vi "FRC-TrajLib-geometry-sample.vi"() -> ()   [LabVIEW 2019]
uses:
  _misc/ROBOT_PICTURE.ctl
  <vilib>/Rock Robotics/WPI/ThirdParty/JAS_Junk/TrajLib/POSE2D.ctl
  <vilib>/Rock Robotics/WPI/ThirdParty/JAS_Junk/TrajLib/TRANSLATION2D.ctl
  <vilib>/Rock Robotics/WPI/ThirdParty/JAS_Junk/TrajLib/ROTATION2D.ctl
  <vilib>/Rock Robotics/WPI/ThirdParty/JAS_Junk/TrajLib/Rotation2d_CreateAngle.vi
  <vilib>/Rock Robotics/WPI/ThirdParty/JAS_Junk/TrajLib/Translation2d_Create.vi
  <vilib>/Rock Robotics/WPI/ThirdParty/JAS_Junk/TrajLib/Transform2d_Create_PosePose.vi
  <vilib>/Rock Robotics/WPI/ThirdParty/JAS_Junk/TrajLib/Pose2d_New_TRRO.vi
  <vilib>/Rock Robotics/WPI/ThirdParty/JAS_Junk/TrajLib/Util_CalcDist.vi
  <vilib>/Rock Robotics/WPI/ThirdParty/JAS_Junk/TrajLib/Rotation2d_UnaryMinus.vi
  <vilib>/Rock Robotics/WPI/ThirdParty/JAS_Junk/TrajLib/Translation2d_RotateBy.vi
  <vilib>/Rock Robotics/WPI/ThirdParty/JAS_Junk/TrajLib/Translation2d_Minus.vi
  <vilib>/Rock Robotics/WPI/ThirdParty/JAS_Junk/TrajLib/Rotation2d_Minus.vi
  <vilib>/Rock Robotics/WPI/ThirdParty/JAS_Junk/TrajLib/Rotation2d_RotateBy.vi
  <vilib>/picture/pixmap.llb/Flatten Pixmap.vi
  <vilib>/picture/pictutil.llb/Create Mask.vi
  <vilib>/picture/picture.llb/Draw Flattened Pixmap.vi
  <vilib>/Rock Robotics/WPI/ThirdParty/JAS_Junk/TrajLib/Trajectory_Library.lvlib
panel:
  in  "Tab Control":enum32{"FIeld", "Additional Data"}(tab)
  out "Robot":T1
  out "BALL":bool=TRUE
  out "Robot POSE":T2 {"ROTATION"."SIN" format="%13.4f"; "ROTATION"."COS" format="%13.4f"; "ROTATION"."VALUE" format="%13.4f"; "TRANSLATION"."Y" format="%14.3f"; "TRANSLATION"."X" format="%14.3f"}
  out "Ball POSE":T2 {"ROTATION"."SIN" format="%13.4f"; "ROTATION"."COS" format="%13.4f"; "ROTATION"."VALUE" format="%13.4f"; "TRANSLATION"."Y" format="%14.3f"; "TRANSLATION"."X" format="%14.3f"}
  out "Pose Ball Relative to Robot":T2 {"ROTATION"."SIN" format="%13.4f"; "ROTATION"."COS" format="%13.4f"; "ROTATION"."VALUE" format="%13.4f"; "TRANSLATION"."Y" format="%14.3f"; "TRANSLATION"."X" format="%14.3f"}
  out "Angle To Ball (Degrees)":dbl
  out "Distance To Ball (Inches)":dbl
  in  "Y  INCHES - BALL":dbl=150.0
  in  "X INCHES - BALL":dbl=200.0
  in  "ORIENTATION - DEG":dbl=42.0
  in  "Y  INCHES":dbl=150.0
  in  "X INCHES":dbl=46.0
  # "Geometry Sample"
  # "ROBOT"
  # "BALL"
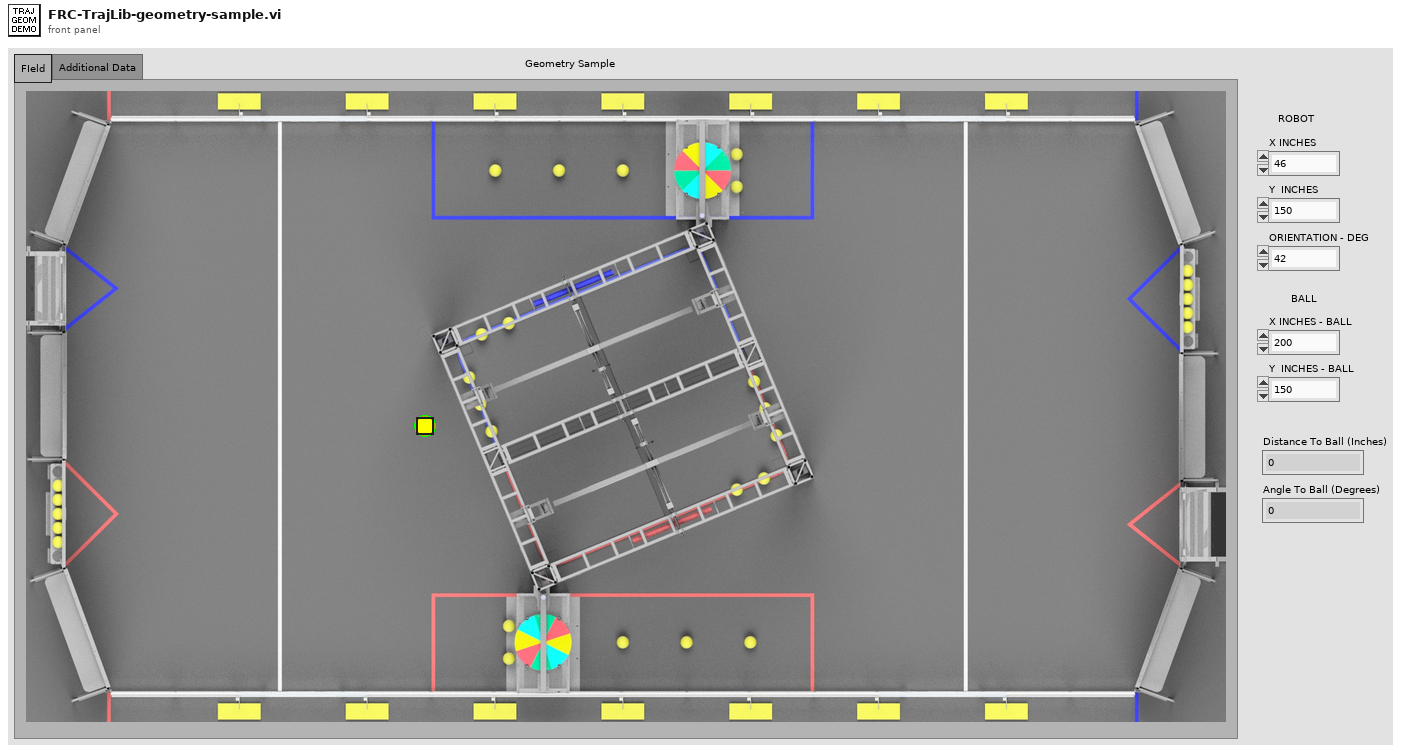
[diagram p1: front panel]
types:
  T1 = typedef "ROBOT_PICTURE.ctl" = picture
  T2 = typedef "Trajectory_Library.lvlib/POSE2D.ctl" = cluster{"TRANSLATION":T3, "ROTATION":T4}
  T3 = typedef "Trajectory_Library.lvlib/TRANSLATION2D.ctl" = cluster{"X":dbl, "Y":dbl}
  T4 = typedef "Trajectory_Library.lvlib/ROTATION2D.ctl" = cluster{"VALUE":dbl, "COS":dbl, "SIN":dbl}
  T5 = typedef "Rotated_Picture_TypeDef.ctl" = cluster{"ONE-8-bit pixmap":u8[][], "Two-Array":cdb[][], "Three-Numeric":i32, "Four-Numeric":i32, "Five-Numeric":cdb, "Six-colors":u32[], "Seven-new element/subarray":u32, "Eight-Cluster":cluster{"[0]":i32, "[1]":i32}}
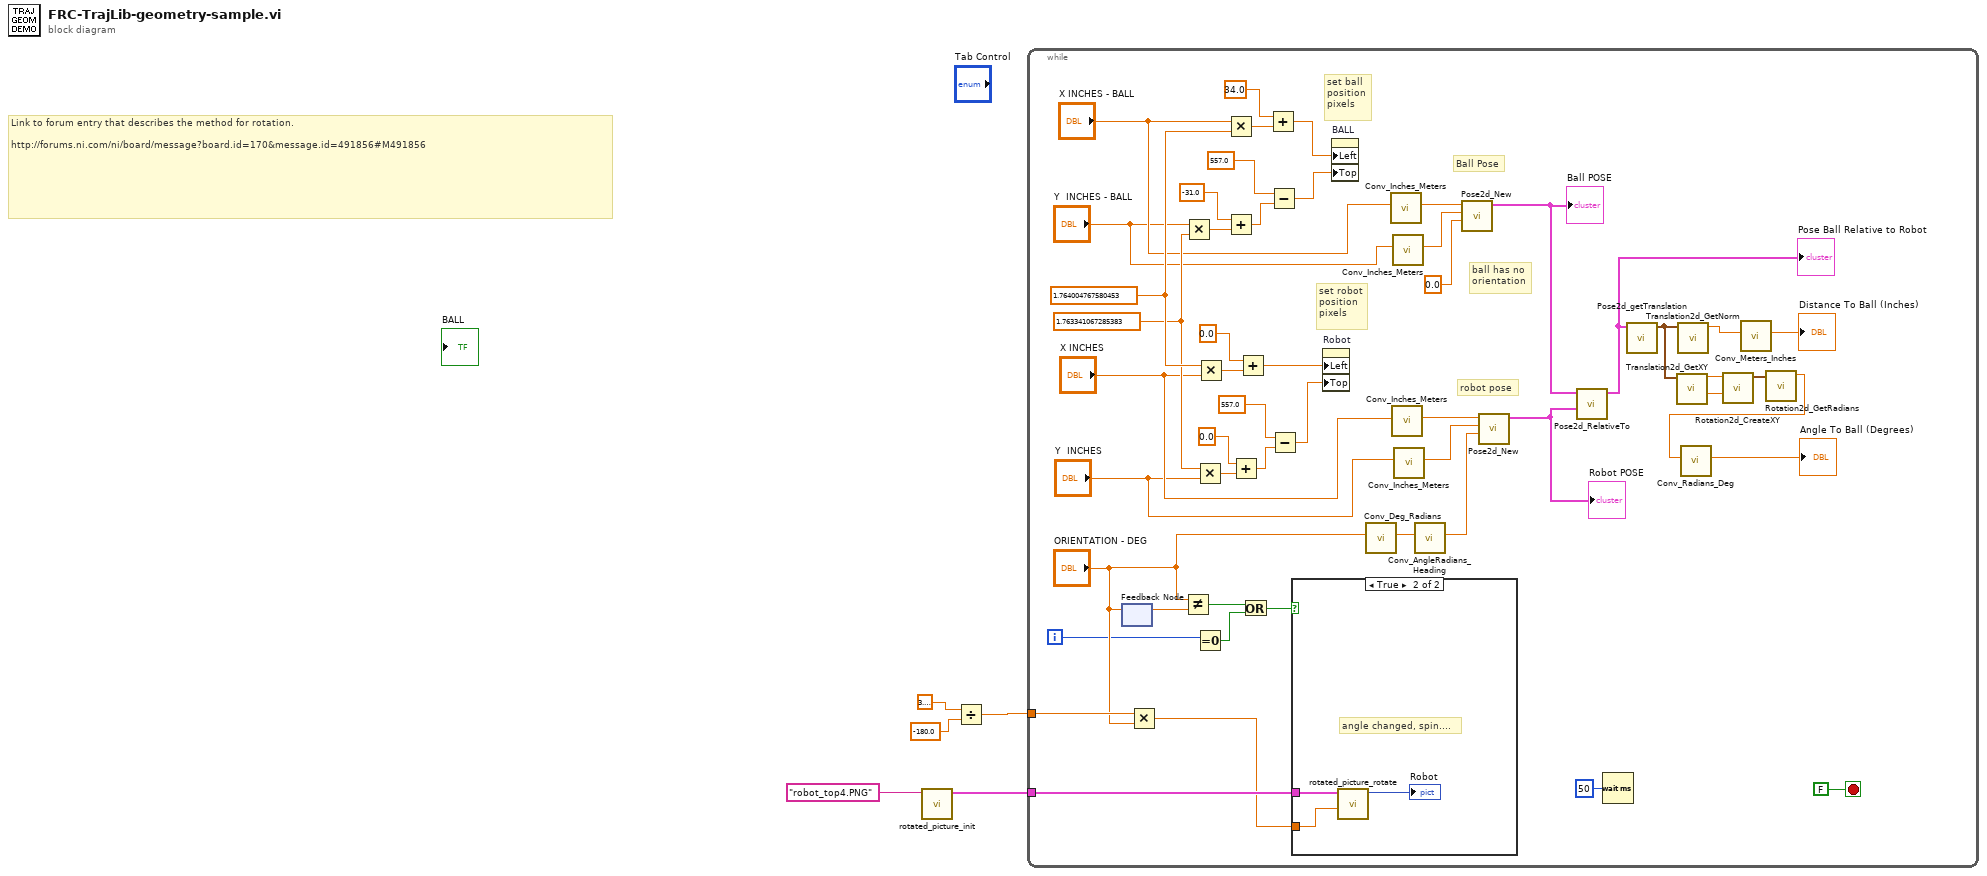
[diagram p0: block diagram]
diagram:
  # "Link to forum entry that describes the method for rotation.\n\nhttp://forums.ni.com/ni/board/message?board.id=170&message.id=491856#M491856"
  n1 = call "rotated_picture_init.vi"("Picture FIle Name"="robot_top4.PNG" ("name or relative path")) -> ("RotatedPictureInfo"=w1:T5)  [unwired: 10 in]
  n2 = Divide(x=3.141592653589793, y=-180.0 ("value")) -> (x/y=w3:dbl)
  n3 = while {
    tunnel: w3 -> [w56]
    tunnel: w1 -> [w55]
    i -> [w20]
    stop <- FALSE stop-if-true
    w33 = 1.763341067285383
    w40 = 1.764004767580453
    # "ball has no\norientation"
    # "robot pose"
    # "Ball Pose"
    # "set robot\nposition\npixels"
    # "set ball \nposition\npixels"
    n4 = feedback-in #1("ORIENTATION - DEG") -> ()
    n5 = feedback #1() -> (w51:dbl)  [unwired: 1 in]
    n6 = Multiply(x=w56, y="ORIENTATION - DEG") -> (x*y=w53:dbl)
    n7 = Not Equal?(x="ORIENTATION - DEG", y=w51) -> (x != y?=w22:bool)
    n8 = Multiply(x="Y  INCHES - BALL", y=w33) -> (x*y=w38:dbl)
    n9 = Multiply(x=w33, y="Y  INCHES") -> (x*y=w48:dbl)
    n10 = Equal To 0?(x=w20) -> (x = 0?=w21:bool)
    n11 = Multiply(x=w40, y="X INCHES") -> (x*y=w50:dbl)
    n12 = Multiply(x="X INCHES - BALL", y=w40) -> (x*y=w42:dbl)
    n13 = Add(x=-31.0, y=w38) -> (x+y=w35:dbl)
    n14 = Add(x=0.0, y=w48) -> (x+y=w44:dbl)
    n15 = Add(x=0.0, y=w50) -> (x+y=w45:dbl)
    n16 = Or(x=w22, y=w21) -> (x .or. y?=w23:bool)
    n17 = Add(x=34.0, y=w42) -> (x+y=w39:dbl)
    n18 = Subtract(x=557.0, y=w35) -> (x-y=w34:dbl)
    n19 = Subtract(x=557.0, y=w44) -> (x-y=w43:dbl)
    n20 = case shown="True" w23 {
      tunnel: w55 -> [_ w58]
      tunnel: w53 -> [_ w57]
      frame False {
        # "Leave as is..."
      }
      frame True {
        # "angle changed, spin...."
        n21 = call "rotated_picture_rotate.vi"("Angle"=w57, "RotatedPictureInfo"=w58) -> ("new picture"=→"Robot":picture)  [unwired: 9 in]
      }
    }
    n22 = property on="Robot" class="Pict (strict)"("Left"=w45, "Top"=w43) -> ()  [unwired: 2 in, 2 out]
    n23 = property on="BALL" class="Bool (strict)"("Left"=w39, "Top"=w34) -> ()  [unwired: 2 in, 2 out]
    n24 = call <vilib>:"Conv_Deg_Radians.vi"("Degress"="ORIENTATION - DEG") -> ("Radians"=w29:dbl)  [unwired: 10 in]
    n25 = call <vilib>:"Conv_Inches_Meters.vi"("INCH"="X INCHES - BALL") -> ("Meters"=w19:dbl)  [unwired: 10 in]
    n26 = call <vilib>:"Conv_Inches_Meters.vi"("INCH"="X INCHES") -> ("Meters"=w28:dbl)  [unwired: 10 in]
    n27 = call <vilib>:"Conv_Inches_Meters.vi"("INCH"="Y  INCHES - BALL") -> ("Meters"=w18:dbl)  [unwired: 10 in]
    n28 = call <vilib>:"Conv_Inches_Meters.vi"("INCH"="Y  INCHES") -> ("Meters"=w27:dbl)  [unwired: 10 in]
    n29 = call <vilib>:"Conv_AngleRadians_Heading.vi"("Radians"=w29) -> ("Heading"=w24:dbl)  [unwired: 10 in]
    n30 = call <vilib>:"Pose2d_New.vi"("Heading"=0.0 ("x"), "Y"=w18, "X"=w19) -> ("out POSe"=w15:T2)  [unwired: 8 in]
    "Ball POSE" <- w15
    n31 = call <vilib>:"Pose2d_New.vi"("Heading"=w24, "Y"=w27, "X"=w28) -> ("out POSe"=w14:T2)  [unwired: 8 in]
    "Robot POSE" <- w14
    n32 = call <vilib>:"Pose2d_RelativeTo.vi"("other POSE"=w14, "in POSE"=w15) -> ("out POSE"=w16:T2)  [unwired: 9 in]
    "Pose Ball Relative to Robot" <- w16
    n33 = Wait (ms)(milliseconds to wait=u32 50) -> ()  [unwired: 1 out]
    n34 = call <vilib>:"Pose2d_getTranslation.vi"("in POSE"=w16) -> ("outTRANSLATION"=w13:T3)  [unwired: 10 in]
    n35 = call <vilib>:"Translation2d_GetXY.vi"("In Translation"=w13) -> ("Y"=w11:dbl, "X"=w12:dbl)  [unwired: 9 in]
    n36 = call <vilib>:"Translation2d_GetNorm.vi"("In Translation"=w13) -> ("Norm"=w7:dbl)  [unwired: 10 in]
    n37 = call <vilib>:"Rotation2d_CreateXY.vi"("Y or sine"=w11, "X or  cosine"=w12) -> ("ROTATION"=w10:T4)  [unwired: 9 in]
    n38 = call <vilib>:"Conv_Meters_Inches.vi"("Meters"=w7) -> ("Inches"=→"Distance To Ball (Inches)":dbl)  [unwired: 10 in]
    n39 = call <vilib>:"Rotation2d_GetRadians.vi"("in ROTATION"=w10) -> ("AngleRadians"=w9:dbl)  [unwired: 10 in]
    n40 = call <vilib>:"Conv_Radians_Deg.vi"("Radians"=w9) -> ("Degrees"=→"Angle To Ball (Degrees)":dbl)  [unwired: 10 in]
  }
